vi "pr-ranking.vi"(2 "element":dbl, 3 "Database Array":dbl[](array[numeric])) -> (0 "Database Size":i32, 1 "PR Value":dbl)   [LabVIEW 2012]
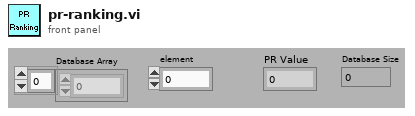
[diagram p1: front panel]
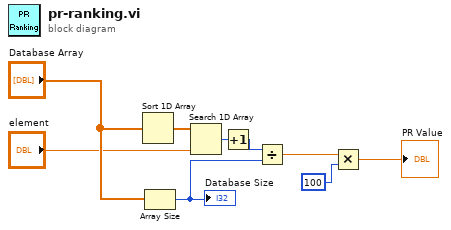
[diagram p0: block diagram]
diagram:
  n1 = Sort 1D Array(array="Database Array") -> (sorted array=w1:dbl[])
  n2 = Array Size(array="Database Array") -> (size(s)=w2:i32)
  "Database Size" <- w2
  n3 = Search 1D Array(1D array=w1, element="element") -> (index of element=w3:i32)  [unwired: 1 in]
  n4 = Increment(x=w3) -> (x+1=w4:i32)
  n5 = Divide(x=w4, y=w2) -> (x/y=w5:dbl)
  n6 = Multiply(x=w5, y=100) -> (x*y=→"PR Value":dbl)
